vi "CommandPSNumber (SubVI).vi"(9 "BUFFER NUMBER(1~8)":u8, 11 "data in":string="BLOAD,") -> (1 "COMMAND (Hex)":string, 3 "NUMBER":u8)   [LabVIEW 2019, in "SR_2000.lvlib"]
uses:
  SR_2000.lvlib
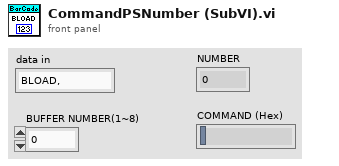
[diagram p1: front panel]
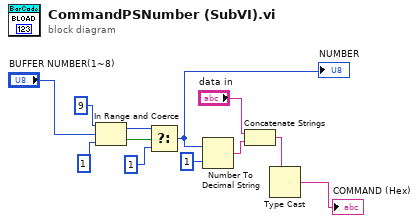
[diagram p0: block diagram]
diagram:
  n1 = In Range and Coerce(upper limit=u8 9, x="BUFFER NUMBER(1~8)", lower limit=u8 1 ("y")) -> (coerced(x)=w5:u8, In Range?=w4:bool)
  n2 = Select(t=w5, s=w4, f=u8 1) -> (s? t:f=w12:u8)
  "NUMBER" <- w12
  n3 = Number To Decimal String(number=w12, width (-)=i16 1) -> (decimal integer string=w8:string)
  n4 = Concatenate Strings("data in", w8) -> (w10:string)
  n5 = Type Cast(x=w10) -> (*(type *) &x=→"COMMAND (Hex)":string)  [unwired: 1 in]
